vi "new orbit fit available.vi"(8 "error in (no error)":errorcluster, 11 "timeout in ms (-1)":i32=20) -> (0 "error out":errorcluster, 2 "new fit available":bool, 3 "orbit fit":T1)   [LabVIEW 2017]
uses:
  typedefs/orbit parameters with crossing info.ctl
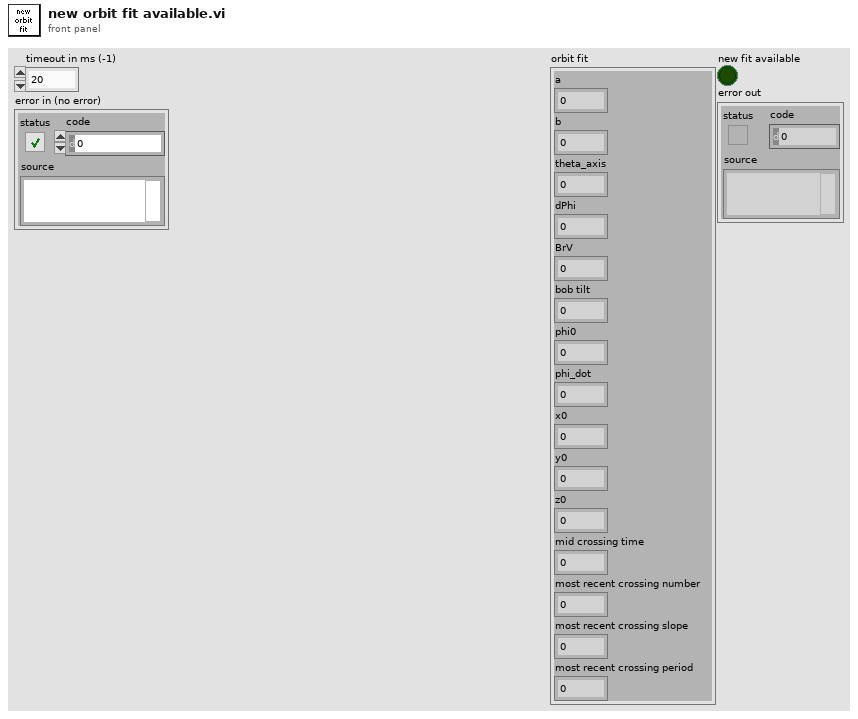
[diagram p1: front panel]
types:
  T1 = typedef "orbit parameters with crossing info.ctl" = cluster{"a":dbl, "b":dbl, "theta_axis":dbl, "dPhi":dbl, "BrV":dbl, "bob tilt":dbl, "phi0":dbl, "phi_dot":dbl, "x0":dbl, "y0":dbl, "z0":dbl, "mid crossing time":dbl, "most recent crossing number":dbl, "most recent crossing slope":dbl, "most recent crossing period":dbl}
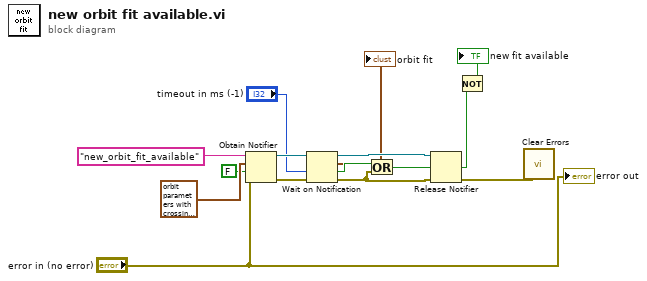
[diagram p0: block diagram]
diagram:
  n1 = Obtain Notifier(name (unnamed)="new_orbit_fit_available", notification data type=T1 {"a"=111.61721095479838, "b"=0.8551138209440372, "theta_axis"=1.6616164149353057, "dPhi"=0.03749673892736358, "BrV"=-1111.1335018896502, "bob tilt"=-0.07911968949071246, "phi0"=3.654809006711329, "phi_dot"=1.002646884100928, "x0"=0.7835120639470753, "y0"=-0.7395215577094556, "z0"=49.927016248136525, "mid crossing time"=582.8819199999999, "most recent crossing number"=505.0, "most recent crossing slope"=69.12255706686331, "most recent crossing period"=2.2081920000000537} ("orbit parameters"), create if not found? (T)=FALSE, error in (no error)="error in (no error)") -> (notifier out=w10:refnum<notifier>, error out=w11:errorcluster)  [unwired: 1 out]
  n2 = Wait on Notification(notifier=w10, timeout in ms (-1)="timeout in ms (-1)", error in (no error)=w11) -> (notifier out=w6:refnum<notifier>, notification=→"orbit fit":T1, timed out?=w8:bool, error out=w7:errorcluster)  [unwired: 1 in]
  n3 = Or(x=w8, y=w7) -> (x .or. y?=w3:bool)
  n4 = Release Notifier(notifier=w6, error in (no error)=w7) -> (error out=w5:errorcluster)  [unwired: 1 in, 2 out]
  n5 = Not(x=w3) -> (.not. x?=→"new fit available":bool)
  n6 = call <vilib>:"Clear Errors.vi"("error in (no error)"=w5) -> ()  [unwired: 5 in, 2 out]
  "error out" <- "error in (no error)"
